vi "未命名 2.vi"() -> ()   [LabVIEW 2017]
panel:
  out "波形图":dbl[](graph)
  out "x*y":dbl[](array[numeric])
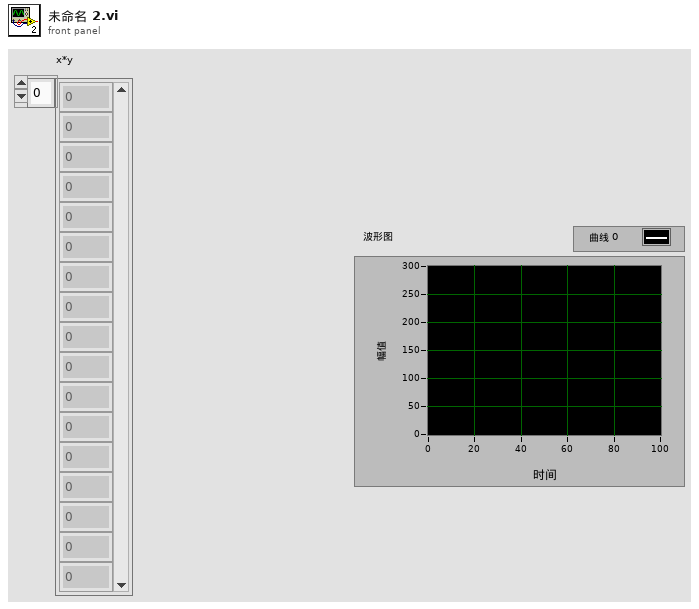
[diagram p1: front panel]
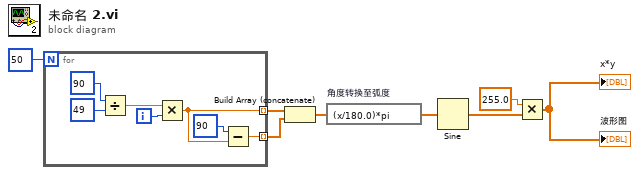
[diagram p0: block diagram]
diagram:
  n1 = for {
    N: 50 -> [_]
    tunnel: [w9] -> w4 mode=indexing
    tunnel: [w10] -> w3 mode=indexing
    i -> [w12]
    n2 = Divide(x=90, y=49) -> (x/y=w13:dbl)
    n3 = Multiply(x=w13, y=w12) -> (x*y=w10:dbl)
    n4 = Subtract(x=90, y=w10) -> (x-y=w9:dbl)
  }
  n5 = Build Array (concatenate)(w3, w4) -> (w2:dbl[])
  n6 = expression code="(x/180.0)*pi" "角度转换至弧度"(w2) -> (w5:dbl[])
  n7 = Sine(x=w5) -> (sin(x)=w6:dbl[])
  n8 = Multiply(x=255.0, y=w6) -> (x*y=→"x*y" →"波形图":dbl[])
